vi "niFPGA Convert LUT Val to Hanning Coeff.vi"(0 "LUT value":u32, 9 "fractional index":fxp<+,16,0>) -> (6 "Hanning coefficient":fxp<+,17,0> format="%.17g")   [LabVIEW 2017]
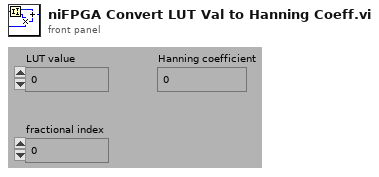
[diagram p1: front panel]
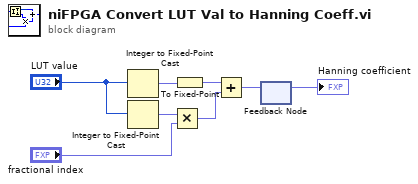
[diagram p0: block diagram]
diagram:
  n1 = Integer to Fixed-Point Cast(integer="LUT value") -> (fixed-point=w7:fxp<+,32,0>)  [unwired: 1 in]
  n2 = Integer to Fixed-Point Cast(integer="LUT value") -> (fixed-point=w4:fxp<+/-,13,-7>)  [unwired: 1 in]
  n3 = Multiply(x=w4, y="fractional index") -> (x*y=w8:fxp<+/-,29,-7>)
  n4 = To Fixed-Point(number=w7) -> (fixed-point=w6:fxp<+,19,0>)  [unwired: 1 in]
  n5 = Add(x=w6, y=w8) -> (x+y=w2:fxp<+,17,0>)
  n6 = feedback-in #1(w2) -> ()
  n7 = feedback #1() -> (→"Hanning coefficient":fxp<+,17,0>)  [unwired: 1 in]
